vi "C867_Stop.vi"(8 "error in":errorcluster caption="entrée d'erreur", 11 "ID":i32) -> (0 "error out":errorcluster caption="sortie d'erreur")   [LabVIEW 2026]
uses:
  C867-VIs/Low Level/PI_GCS2_DLL_x64.dll
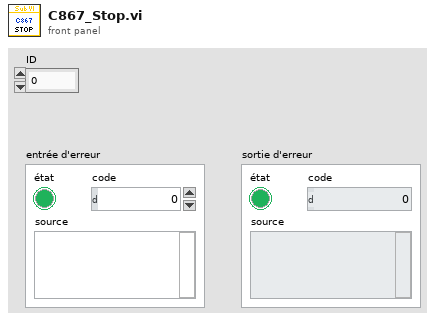
[diagram p1: front panel]
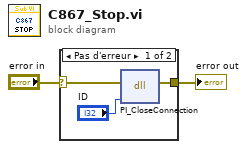
[diagram p0: block diagram]
diagram:
  n1 = case shown="Pas d'erreur" "error in" {
    selector: "error in" -> [w3 w6]
    tunnel: [w5 w6] -> w1
    frame No Error {
      n2 = dll-call lib="D:/SEBASTIEN/GitHub/LABVIEW-Useful-codes/Device_control/PC-C867-IO Control/v0.2/SubVI/PI-C867/C867-VIs/Low Level/PI_GCS2_DLL_x64.dll" fn="PI_CloseConnection"(error in=w3, "ID"="ID") -> (error out=w5:errorcluster)  [unwired: 4 in, 1 out]
    }
    frame Error {
    }
  }
  "error out" <- w1
